vi "PH_Beckhoff_PP_PU.HV Meas Scaling.vi"(4 "Devider [Hz/kV]":dbl=184.21, 5 "Subtractor [Hz]":dbl=15.79, 6 "Period Time [s]":dbl=0.05, 7 "Beckhoff value":u32) -> (0 "Spannung [V]":i32)   [LabVIEW 2014, in "PH_Beckhoff_PP_PU.lvlib"]
doc: "This VI scales the Beckhoff value to calculate the voltage; after a linear regression, the value is rounded to multiples of 100."
uses:
  PH_Beckhoff_PP_PU.lvlib
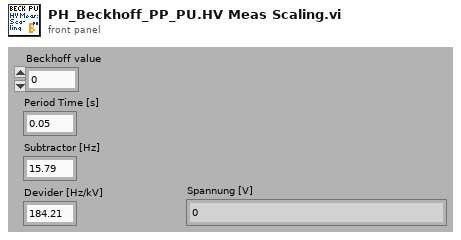
[diagram p1: front panel]
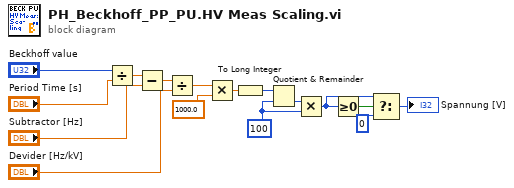
[diagram p0: block diagram]
diagram:
  w6 = 100 ("y")
  n1 = Divide(x="Beckhoff value", y="Period Time [s]") -> (x/y=w11:dbl)
  n2 = Subtract(x=w11, y="Subtractor [Hz]") -> (x-y=w12:dbl)
  n3 = Divide(x=w12, y="Devider [Hz/kV]") -> (x/y=w16:dbl)
  n4 = Multiply(x=w16, y=1000.0) -> (x*y=w9:dbl)
  n5 = To Long Integer(number=w9) -> (32bit integer=w5:i32)
  n6 = Quotient & Remainder(x=w5, y=w6) -> (floor(x/y)=w7:i32)  [unwired: 1 out]
  n7 = Multiply(x=w7, y=w6) -> (x*y=w1:i32)
  n8 = Greater Or Equal To 0?(x=w1) -> (x >= 0?=w4:bool)
  n9 = Select(t=w1, s=w4, f=0) -> (s? t:f=→"Spannung [V]":i32)
